vi "get Spec String.vi"(8 "error in (no error)":errorcluster) -> (0 "error out":errorcluster, 3 "function return":string)   [LabVIEW 2019, in "libSpecValiReader.lvlib"]
doc: "const char* getSpecString();"
uses:
  libSpecValiReader.lvlib
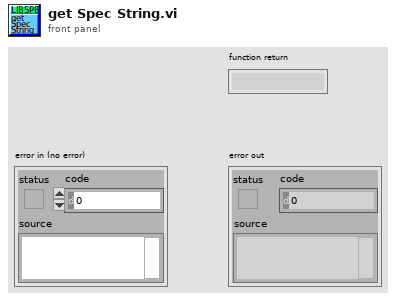
[diagram p1: front panel]
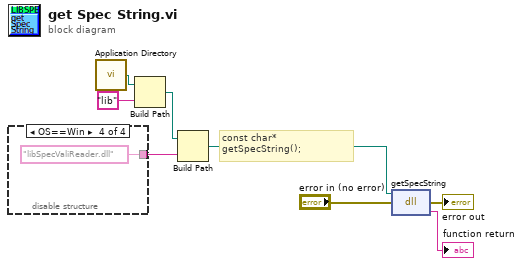
[diagram p0: block diagram]
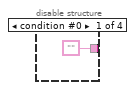
[diagram p2: hidden frame]
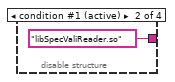
[diagram p3: hidden frame]
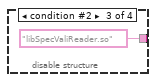
[diagram p4: hidden frame]
diagram:
  # "const char* getSpecString();"
  n1 = disable-structure shown="OS==Win" {
    disable-tunnel: ["" "libSpecValiReader.so" ("name or relative path") "libSpecValiReader.so" ("name or relative path") "libSpecValiReader.dll" ("name or relative path")] -> w2
    frame condition #0 {
    }
    frame condition #1 (active) {
    }
    frame condition #2 {
    }
    frame condition #3 {
    }
  }
  n2 = call <vilib>:"Application Directory.vi"() -> ("Application Directory"=w5:path)
  n3 = Build Path(base path=w5, name or relative path="lib") -> (appended path=w3:path)
  n4 = Build Path(base path=w3, name or relative path=w2) -> (appended path=w1:path)
  n5 = dll-call lib="home/paul/Schreibtisch/Biogas_plant_setup/LabView/lib/libSpecValiReader/libSpecValiReader.*" fn="getSpecString"(path in=w1, error in="error in (no error)") -> (error out=→"error out":errorcluster, "return type"=→"function return":string)  [unwired: 1 in, 1 out]
